vi "J1939 Workspace Tool.vi"() -> ()   [LabVIEW 2019, in "J1939 Workspace Tool.lvlib"]
uses:
  J1939 Workspace Tool.lvlib
  NationalInstruments.VeriStand.SystemStorage
  Workspace Shared/Types/UI.StateVariables.ctl
  <vilib>/NI VeriStand/Display Template Support/DisplayTemplateSupport.llb/enum_Display Template Handler Minimal To Widget Msg.ctl
  <vilib>/NI VeriStand/Execution/Workspace/SystemStateRegEventRef.ctl
  <vilib>/NI VeriStand/Execution/Workspace/Target State Info.ctl
  <vilib>/NI VeriStand/Execution/Workspace/Target State.ctl
  Shared/Types/Private Data.ctl
  <vilib>/NI/STM/TCP/TCP Connection Info.ctl
  <vilib>/NI/STM/SubVIs/MetaDataElement.ctl
  Shared/Types/Error Cluster.ctl
  Shared/Types/Error Types.ctl
  <vilib>/NI VeriStand/Display Template Support/DisplayTemplateSupport.llb/enum_Display Template Handler Minimal To Workspace.ctl
  <vilib>/NI VeriStand/Execution/Workspace/WorkspaceAPI.ctl
  <vilib>/NI VeriStand/Execution/Workspace/SystemStateEventRef.ctl
  Workspace Shared/Types/UI.Refs.ctl
  <vilib>/Utility/miscctls.llb/LVStringsAndValuesArrayTypeDef_U8.ctl
  Shared/J1939 Utilities/SubVIs/Convert CAN Arb ID to J1939 ID.vi
  <vilib>/NI VeriStand/Execution/Workspace/NI_VS Workspace ExecutionAPI.lvlib
  Shared/J1939 Utilities/J1939 Utilities.lvlib
  Shared/J1939 Addon Shared.lvlib
  <vilib>/NI/STM/NI STM.lvlib
  Workspace Shared/J1939 Workspace Shared.lvlib
  NationalInstruments.VeriStand.ClientAPI
panel:
  in  "NIVS.Workspace Event":refnum<event-registration>
  in  "NIVS.Gateway IP Address":string
  in  "NIVS.System Definition Root":refnum<k24>
  in  "Tab Control":enum32{"DTCs", "Custom RQST", "RAW FRAME"}(tab)
  in  "Refresh Continuous":bool
  in  "Clear DTC":bool
  in  "Refresh DTCs":bool
  in  "DTCs":i32(listbox)
  in  "Addresses":string(tree)
  in  "Refresh Addresses":bool
  out "Response":string
  in  "Request":bool
  in  "PGN":u32 format="%.0x"
  in  "DA":u8(ring)
  in  "Clear Array":bool
  in  "RAW":bool
  out "Priority":u8 format="%02x"
  out "SA":u8 format="%02x"
  out "PGN":u32 format="%06x"
  in  "Identifier":u32 format="%08x"
  in  "Data":u8[](array[numeric])=[0, 0, 0, 0, 0, 0, 0, 0] format="%.0x"
  out "Device":string
  in  "Errors":bool
  # "This is the root reference to the active System Definition file. You could use this to read the configuration or populate a tree with channels. You are free to close this reference, but it will be closed for you if you don't."
  # "The SystemStorageUI .NET assembly provides controls to display data configured in the System Definition file."
  # "This is the IP Address of the VeriStand Gateway to which the Workspace is connected. Use this to open all the .NET Manager references. Usually the Gateway is running on localhost, but it could be running on a neighbor's machine."
  # "This registered string User Event is used to help instruct your tool to shut down when the Workspace is closing."
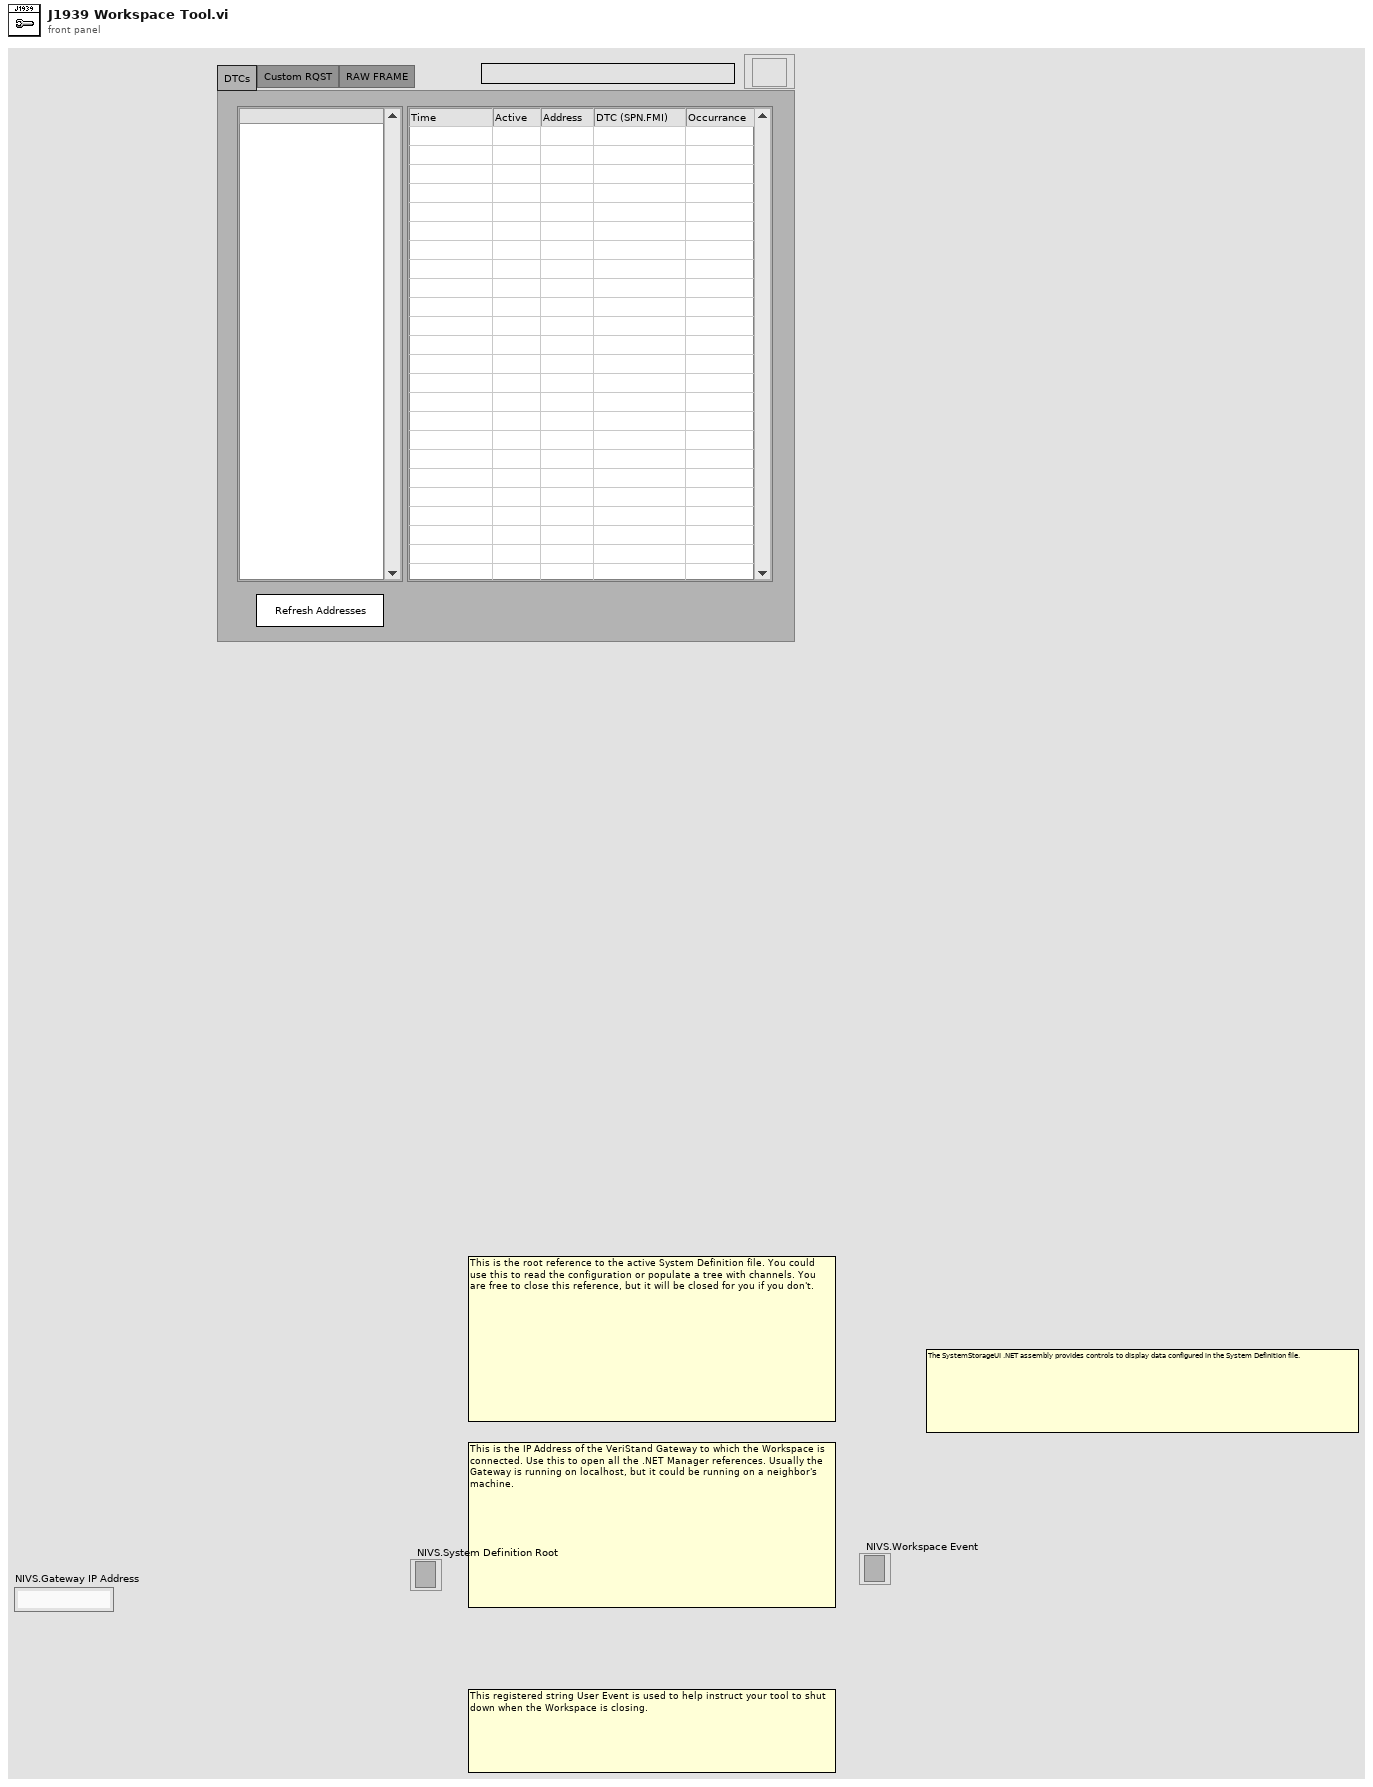
[diagram p1: front panel]
types:
  T1 = typedef "J1939 Addon Shared.lvlib/Private Data.ctl" = cluster{"PGN":u32, "DA":u8, "CD Path":string, "CD IP":string}
  T2 = typedef "J1939 Workspace Shared.lvlib/UI.StateVariables.ctl" = cluster{"NIVS.Gateway IP Address":string, "LaunchConfig.Ref":refnum<user-event>, "Events.Refs":cluster{"LaunchConfig":refnum<event-registration>, "SystemChange":T3, "NIVS.Workspace":refnum<event-registration>}, "State":T1, "TCP.Refs":T4, "Addresses.LUT":variant, "Errors.Q":refnum<queue>, "NIVS.System Definition Root":refnum<k24>, "State.Notifier":refnum<user-event>, "NIVS.Workspace.Ref":T6, "DTCs.Refresh":bool, "NIVS.State.Refs":T7, "UI.Refs":T8, "Workspace.Connected":bool, "DTCs.Timer":u32}
  T3 = typedef "NI_VS Workspace ExecutionAPI.lvlib/SystemStateRegEventRef.ctl" = refnum<event-registration>
  T4 = typedef "NI STM.lvlib/TCP Connection Info.ctl" = cluster{"connection ID":refnum<k5>, "meta data":T5[]}
  T5 = typedef "NI STM.lvlib/MetaDataElement.ctl" = string
  T6 = typedef "NI_VS Workspace ExecutionAPI.lvlib/WorkspaceAPI.ctl" = refnum<k24>
  T7 = typedef "NI_VS Workspace ExecutionAPI.lvlib/SystemStateEventRef.ctl" = cluster{"CustDatRef":refnum<user-event>, "EvtRef":refnum<k27>, "Target State User Event":refnum<user-event>}
  T8 = typedef "J1939 Workspace Shared.lvlib/UI.Refs.ctl" = cluster{"ParentVI":refnum<vi>, "DTCs":refnum<vi>, "Addresses":refnum<vi>, "Device":refnum<vi>, "Data":refnum<vi>, "Identifier":refnum<vi>, "PGN":refnum<vi>, "DA":refnum<vi>, "Refresh Continuous":refnum<vi>, "Errors":refnum<vi>, "Refresh Addresses":refnum<vi>, "Refresh DTCs":refnum<vi>, "Clear DTC":refnum<vi>, "Request":refnum<vi>, "Clear Array":refnum<vi>, "RAW":refnum<vi>}
  T9 = enum8{"Enabled", "Disabled", "Disabled and Grayed Out"}
  T10 = typedef "LVStringsAndValuesArrayTypeDef_U8.ctl" = cluster{"String":string, "Value":u8}[]
  T11 = cluster{"LaunchConfig":refnum<event-registration>, "SystemChange":T3, "NIVS.Workspace":refnum<event-registration>}
  T12 = typedef "enum_Display Template Handler Minimal To Widget Msg.ctl" = enum16{"Stop", "LaunchConfigDialog"}
  T13 = typedef "NI_VS Workspace ExecutionAPI.lvlib/SystemState.ctl" = u8
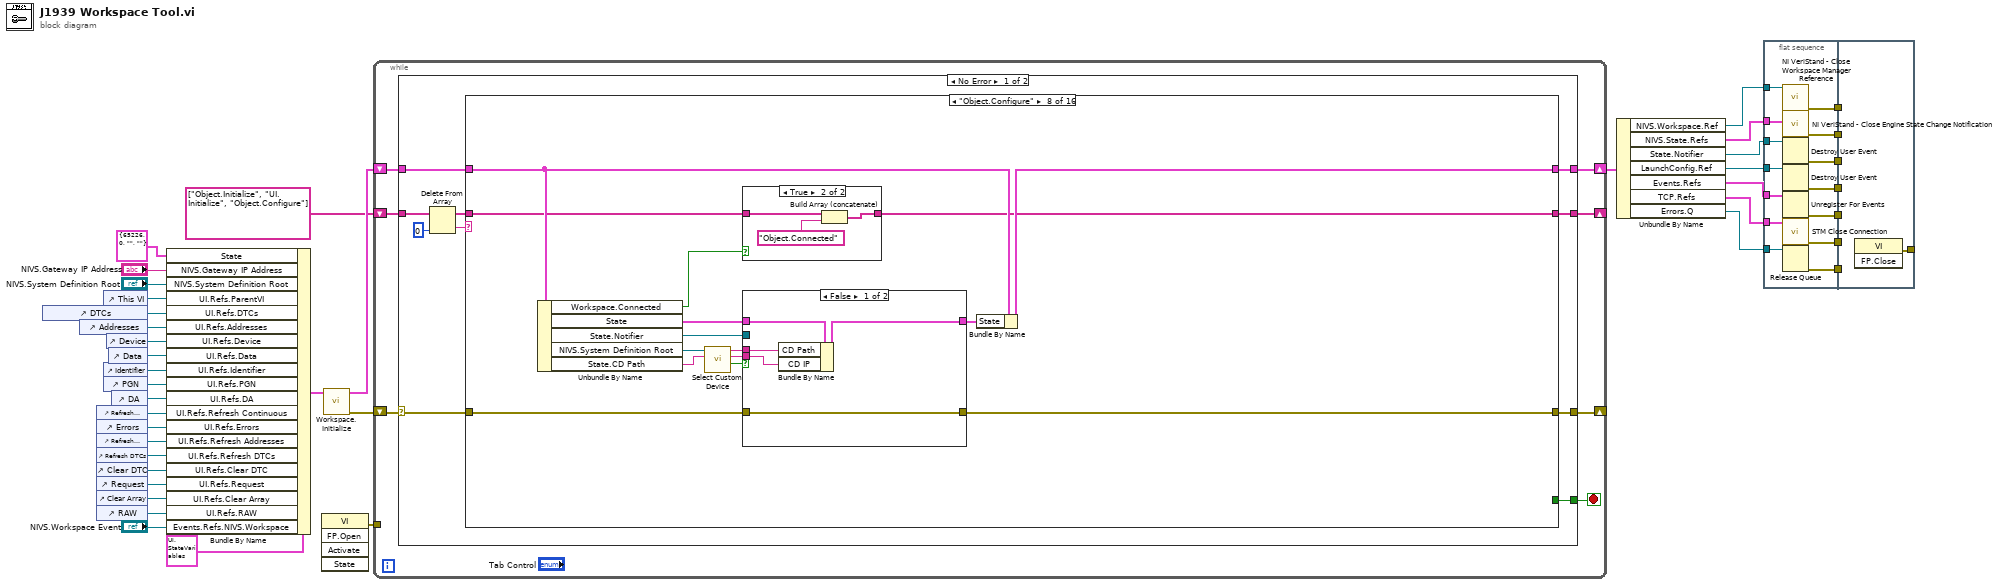
[diagram p0: block diagram]
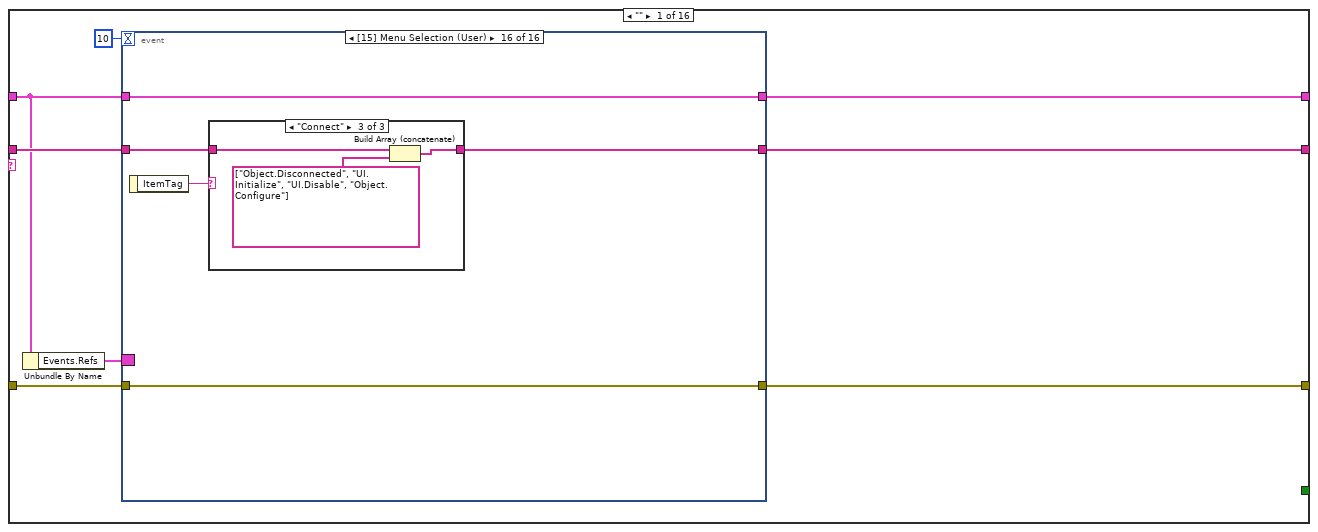
[diagram p2: hidden frame]
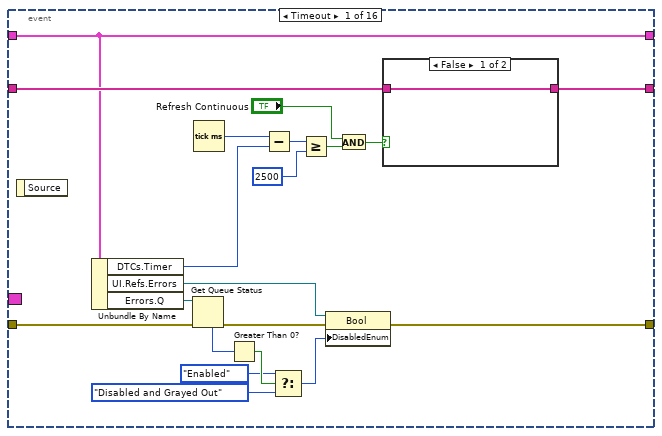
[diagram p3: hidden frame]
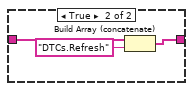
[diagram p4: hidden frame]
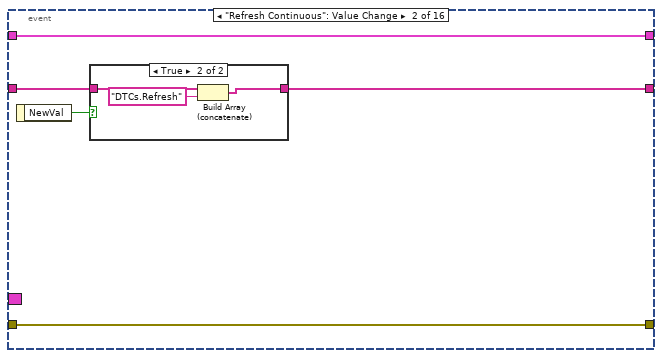
[diagram p5: hidden frame]
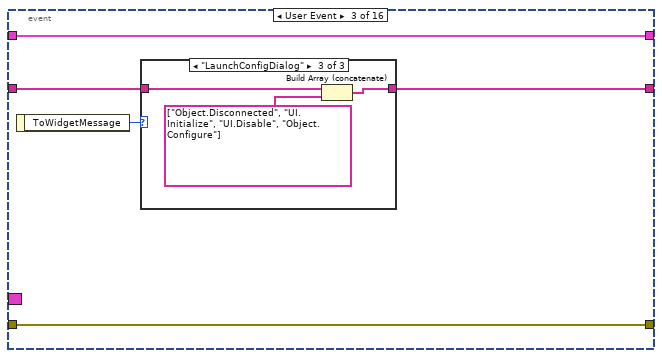
[diagram p7: hidden frame]
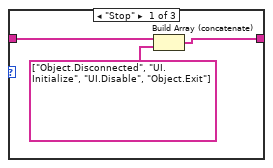
[diagram p8: hidden frame]
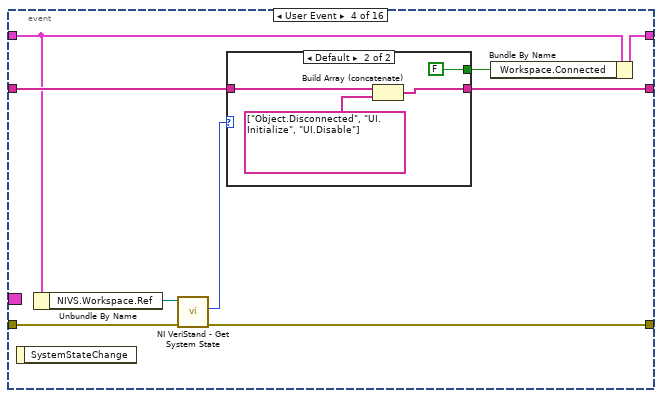
[diagram p10: hidden frame]
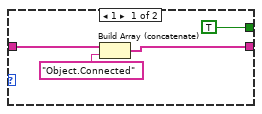
[diagram p11: hidden frame]
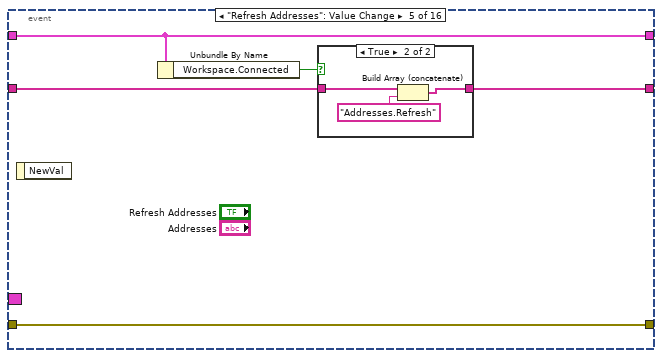
[diagram p12: hidden frame]
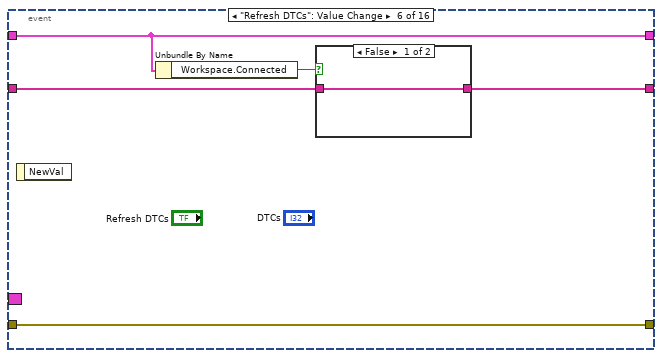
[diagram p14: hidden frame]
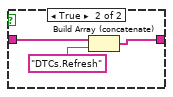
[diagram p15: hidden frame]
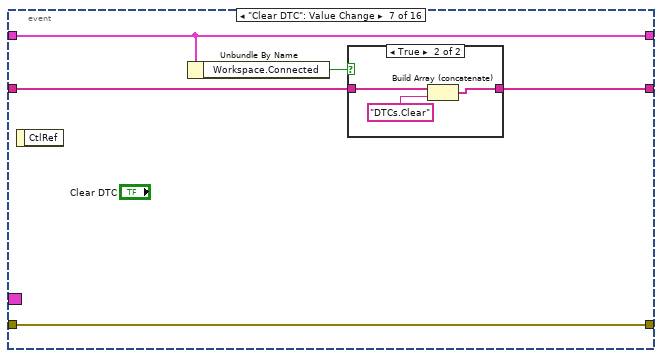
[diagram p16: hidden frame]
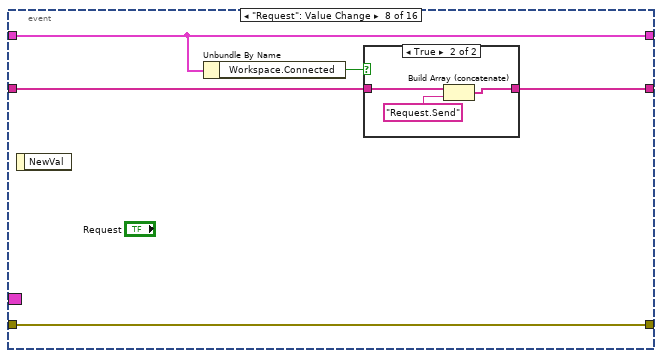
[diagram p18: hidden frame]
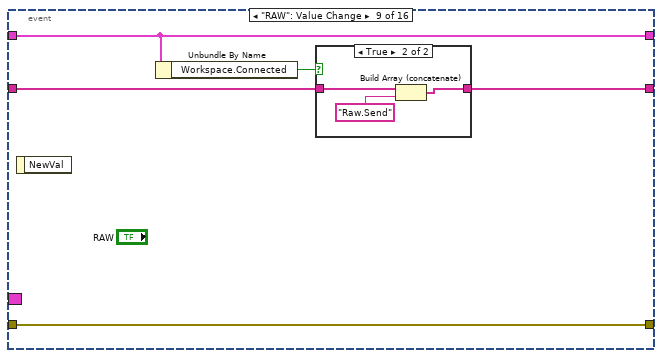
[diagram p20: hidden frame]
diagram:
  n1 = control-ref of="DTCs"() -> (w35:refnum<vi>)
  n2 = control-ref of="Addresses"() -> (w34:refnum<vi>)
  n3 = control-ref of="Refresh Continuous"() -> (w28:refnum<vi>)
  n4 = control-ref of="Errors"() -> (w27:refnum<vi>)
  n5 = control-ref of="Refresh Addresses"() -> (w26:refnum<vi>)
  n6 = control-ref of="Refresh DTCs"() -> (w25:refnum<vi>)
  n7 = control-ref of="Clear DTC"() -> (w24:refnum<vi>)
  n8 = control-ref of="Request"() -> (w23:refnum<vi>)
  n9 = control-ref of="Clear Array"() -> (w22:refnum<vi>)
  n10 = control-ref of="RAW"() -> (w21:refnum<vi>)
  n11 = control-ref of="This VI"() -> (w36:refnum<vi>)
  n12 = control-ref of="Identifier"() -> (w31:refnum<vi>)
  n13 = control-ref of="PGN"() -> (w30:refnum<vi>)
  n14 = control-ref of="Device"() -> (w33:refnum<vi>)
  n15 = control-ref of="Data"() -> (w32:refnum<vi>)
  n16 = control-ref of="DA"() -> (w29:refnum<vi>)
  n17 = Bundle By Name(cluster=T2 {"NIVS.Gateway IP Address"="", "LaunchConfig.Ref"=refnum, "Events.Refs"={"LaunchConfig"=refnum, "SystemChange"=refnum, "NIVS.Workspace"=refnum}, "State"={"PGN"=0, "DA"=0, "CD Path"="", "CD IP"=""}, "TCP.Refs"={"connection ID"=refnum, "meta data"=[]}, "Addresses.LUT"=variant, "Errors.Q"=refnum, "NIVS.System Definition Root"=refnum, "State.Notifier"=refnum, "NIVS.Workspace.Ref"=refnum, "DTCs.Refresh"=FALSE, "NIVS.State.Refs"={"CustDatRef"=refnum, "EvtRef"=refnum, "Target State User Event"=refnum}, "UI.Refs"={"ParentVI"=refnum, "DTCs"=refnum, "Addresses"=refnum, "Device"=refnum, "Data"=refnum, "Identifier"=refnum, "PGN"=refnum, "DA"=refnum, "Refresh Continuous"=refnum, "Errors"=refnum, "Refresh Addresses"=refnum, "Refresh DTCs"=refnum, "Clear DTC"=refnum, "Request"=refnum, "Clear Array"=refnum, "RAW"=refnum}, "Workspace.Connected"=FALSE, "DTCs.Timer"=0}, "State"=T1 {"PGN"=65226, "DA"=0, "CD Path"="", "CD IP"=""} ("Cluster"), "NIVS.Gateway IP Address"="NIVS.Gateway IP Address", "NIVS.System Definition Root"="NIVS.System Definition Root", "UI.Refs.ParentVI"=w36, "UI.Refs.DTCs"=w35, "UI.Refs.Addresses"=w34, "UI.Refs.Device"=w33, "UI.Refs.Data"=w32, "UI.Refs.Identifier"=w31, "UI.Refs.PGN"=w30, "UI.Refs.DA"=w29, "UI.Refs.Refresh Continuous"=w28, "UI.Refs.Errors"=w27, "UI.Refs.Refresh Addresses"=w26, "UI.Refs.Refresh DTCs"=w25, "UI.Refs.Clear DTC"=w24, "UI.Refs.Request"=w23, "UI.Refs.Clear Array"=w22, "UI.Refs.RAW"=w21, "Events.Refs.NIVS.Workspace"="NIVS.Workspace Event") -> (w38:T2)
  n18 = invoke class="VI" method="FP.Open"() -> (error out=w8:errorcluster)  [unwired: 5 in, 4 out]
  n19 = call "Workspace.Initialize.vi"("State"=w38) -> ("error out"=w37:errorcluster, "State"=w20:T2)  [unwired: 9 in]
  n20 = while {
    shift-right: [w46] -> _
    shift-left: w37 -> [w47]
    shift-right: [w42] -> w18
    shift-left: w20 -> [w45]
    shift-right: [w43] -> _
    shift-left: string[] ["Object.Initialize", "UI.Initialize", "Object.Configure"] -> [w44]
    tunnel: w8 -> [_]
    stop <- w48 stop-if-true
    n21 = case shown="No Error" w47 {
      selector: w47 -> [w49 w503]
      tunnel: [w58 FALSE] -> w48
      tunnel: [w50 w501] -> w46
      tunnel: w45 -> [w57 w498]
      tunnel: w44 -> [w55 w499]
      tunnel: [w52 w499] -> w43
      tunnel: [w51 w498] -> w42
      frame No Error {
        n22 = Delete From Array(array=w55, index=0) -> (deleted portion=w54:string, array with subset deleted=w53:string[])  [unwired: 1 in]
        n23 = case shown="\"Object.Configure\"" w54 {
          selector: w54 -> [_ _ _ _ _ _ _ _ _ _ _ _ _ _ _ w493]
          tunnel: [_ _ _ _ _ _ _ _ TRUE _ _ _ _ _ _ _] -> w58
          tunnel: w57 -> [w60 w232 w241 w258 w288 w324 w337 w357 w381 w390 w398 w410 w419 w440 w488 w496]
          tunnel: w53 -> [w64 w239 w251 w267 w295 w316 w340 w354 w382 w391 w399 w406 w435 w456 w490 w497]
          tunnel: [w65 w239 w251 w267 w294 w316 w339 w353 w382 w391 w399 w406 w435 w456 w490 w497] -> w52
          tunnel: [w63 w229 w240 w268 w287 w323 w336 w356 w381 w390 w397 w407 w419 w440 w488 w496] -> w51
          tunnel: [w62 w228 w250 w253 w290 w318 w335 w360 w380 w386 w392 w405 w420 w441 w464 w495] -> w50
          tunnel: w49 -> [w61 w228 w250 w254 w289 w319 w325 w361 w380 w385 w392 w405 w422 w443 w489 w495]
          frame "" {
            n24 = Unbundle By Name(w60) -> ("Events.Refs"=w59:T11)
            n25 = event shown="[15] Menu Selection (User)" {
              selector: w59 -> [_ _ _ _ _ _ _ _ _ _ _ _ _ _ _ _]
              dyn-events: _ -> [_ _ _ _ _ _ _ _ _ _ _ _ _ _ _ _]
              timeout: 10 -> [_ _ _ _ _ _ _ _ _ _ _ _ _ _ _ _]
              tunnel: w60 -> [w75 w94 w104 w114 w132 w140 w147 w158 w167 w176 w185 w189 w196 w206 w211 w220]
              tunnel: [w76 w92 w100 w117 w130 w138 w148 w156 w165 w174 w184 w190 w198 w201 w208 w216] -> w65
              tunnel: w64 -> [w77 w93 w101 w118 w131 w139 w149 w157 w166 w175 w187 w190 w198 w202 w209 w218]
              tunnel: [w75 w94 w104 w113 w132 w140 w147 w158 w167 w176 w185 w189 w196 w206 w211 w220] -> w63
              tunnel: [w69 w95 w103 w119 w133 w142 w151 w160 w169 w178 w186 w188 w197 w205 w210 w219] -> w62
              tunnel: w61 -> [w71 w95 w103 w120 w133 w142 w151 w160 w169 w178 w186 w188 w197 w205 w210 w219]
              event Timeout {
                n26 = event-data() -> ()  [unwired: 2 out]
                n27 = Unbundle By Name(w75) -> ("DTCs.Timer"=w68:u32, "UI.Refs.Errors"=w73:refnum<vi>, "Errors.Q"=w74:refnum<queue>)
                n28 = Get Queue Status(queue=w74, error in (no error)=w71) -> (error out=w72:errorcluster, # elements in queue=w86:i32)  [unwired: 1 in, 6 out]
                n29 = Tick Count (ms)() -> (millisecond timer value=w80:u32)
                n30 = Greater Than 0?(x=w86) -> (x > 0?=w85:bool)
                n31 = Subtract(x=w80, y=w68) -> (x-y=w82:u32)
                n32 = Select(t=T9."Enabled" ("Disabled"), s=w85, f=T9."Disabled and Grayed Out") -> (s? t:f=w70:T9)
                n33 = Greater Or Equal?(x=w82, y=u32 2500) -> (x >= y?=w67:bool)
                n34 = property class="Bool"(reference=w73, error in=w72, "DisabledEnum"=w70) -> (error out=w69:errorcluster)  [unwired: 1 out]
                n35 = And(x="Refresh Continuous", y=w67) -> (x .and. y?=w78:bool)
                n36 = case shown="False" w78 {
                  tunnel: w77 -> [w87 w89]
                  tunnel: [w87 w88] -> w76
                  frame False {
                  }
                  frame True {
                    n37 = Build Array (concatenate)(w89, "DTCs.Refresh" ("NewVal")) -> (w88:string[])
                  }
                }
              }
              event "Refresh Continuous": Value Change {
                n38 = event-data() -> ("NewVal"=w91:bool)  [unwired: 1 out]
                n39 = case shown="True" w91 {
                  tunnel: w93 -> [w96 w98]
                  tunnel: [w96 w97] -> w92
                  frame False {
                  }
                  frame True {
                    n40 = Build Array (concatenate)(w98, "DTCs.Refresh" ("NewVal")) -> (w97:string[])
                  }
                }
              }
              event User Event {
                n41 = event-data() -> ("ToWidgetMessage"=w102:T12)  [unwired: 1 out]
                n42 = case shown="\"LaunchConfigDialog\"" w102 {
                  tunnel: w101 -> [w106 w108 w110]
                  tunnel: [w105 w108 w109] -> w100
                  frame "Stop" {
                    n43 = Build Array (concatenate)(w106, string[] ["Object.Disconnected", "UI.Initialize", "UI.Disable", "Object.Exit"]) -> (w105:string[])
                  }
                  frame Default {
                  }
                  frame "LaunchConfigDialog" {
                    n44 = Build Array (concatenate)(w110, string[] ["Object.Disconnected", "UI.Initialize", "UI.Disable", "Object.Configure"]) -> (w109:string[])
                  }
                }
              }
              event User Event {
                n45 = event-data() -> ()  [unwired: 2 out]
                n46 = Unbundle By Name(w114) -> ("NIVS.Workspace.Ref"=w115:T6)
                n47 = call <vilib>:"NI VeriStand - Get System State.vi"("error in (no error)"=w120, "WorkspaceManager in"=w115) -> ("error out"=w119:errorcluster, "System State"=w116:T13)  [unwired: 5 in, 3 out]
                n48 = case shown="Default" w116 {
                  tunnel: w118 -> [w124 w128]
                  tunnel: [w123 w127] -> w117
                  tunnel: [TRUE FALSE] -> w112
                  frame 1 {
                    # "System state is connected"
                    n49 = Build Array (concatenate)(w124, "Object.Connected") -> (w123:string[])
                  }
                  frame Default {
                    # "System state not connected"
                    n50 = Build Array (concatenate)(w128, string[] ["Object.Disconnected", "UI.Initialize", "UI.Disable"]) -> (w127:string[])
                  }
                }
                n51 = Bundle By Name(cluster=w114, "Workspace.Connected"=w112) -> (w113:T2)
              }
              event "Refresh Addresses": Value Change {
                n52 = event-data() -> ()  [unwired: 2 out]
                n53 = Unbundle By Name(w132) -> ("Workspace.Connected"=w129:bool)
                n54 = case shown="True" w129 {
                  tunnel: w131 -> [w134 w136]
                  tunnel: [w134 w135] -> w130
                  frame False {
                  }
                  frame True {
                    n55 = Build Array (concatenate)(w136, "Addresses.Refresh") -> (w135:string[])
                  }
                }
              }
              event "Refresh DTCs": Value Change {
                n56 = event-data() -> ()  [unwired: 2 out]
                n57 = Unbundle By Name(w140) -> ("Workspace.Connected"=w141:bool)
                n58 = case shown="False" w141 {
                  tunnel: w139 -> [w143 w145]
                  tunnel: [w143 w144] -> w138
                  frame False {
                  }
                  frame True {
                    n59 = Build Array (concatenate)(w145, "DTCs.Refresh") -> (w144:string[])
                  }
                }
              }
              event "Clear DTC": Value Change {
                n60 = event-data() -> ()  [unwired: 2 out]
                n61 = Unbundle By Name(w147) -> ("Workspace.Connected"=w150:bool)
                n62 = case shown="True" w150 {
                  tunnel: w149 -> [w152 w154]
                  tunnel: [w152 w153] -> w148
                  frame False {
                  }
                  frame True {
                    n63 = Build Array (concatenate)(w154, "DTCs.Clear") -> (w153:string[])
                  }
                }
              }
              event "Request": Value Change {
                n64 = event-data() -> ()  [unwired: 2 out]
                n65 = Unbundle By Name(w158) -> ("Workspace.Connected"=w159:bool)
                n66 = case shown="True" w159 {
                  tunnel: w157 -> [w161 w163]
                  tunnel: [w161 w162] -> w156
                  frame False {
                  }
                  frame True {
                    n67 = Build Array (concatenate)(w163, "Request.Send") -> (w162:string[])
                  }
                }
              }
              event "RAW": Value Change {
                n68 = event-data() -> ()  [unwired: 2 out]
                n69 = Unbundle By Name(w167) -> ("Workspace.Connected"=w168:bool)
                n70 = case shown="True" w168 {
                  tunnel: w166 -> [w170 w172]
                  tunnel: [w170 w171] -> w165
                  frame False {
                  }
                  frame True {
                    n71 = Build Array (concatenate)(w172, "Raw.Send") -> (w171:string[])
                  }
                }
              }
              event "Clear Array": Value Change {
                n72 = event-data() -> ()  [unwired: 2 out]
                n73 = Unbundle By Name(w176) -> ("Workspace.Connected"=w177:bool)
                n74 = case shown="True" w177 {
                  tunnel: w175 -> [w179 w181]
                  tunnel: [w179 w180] -> w174
                  frame False {
                  }
                  frame True {
                    n75 = Build Array (concatenate)(w181, "Raw.Clear") -> (w180:string[])
                  }
                }
              }
              event "Addresses": Value Change {
                n76 = event-data() -> ()  [unwired: 2 out]
                n77 = Build Array (concatenate)(w187, "DTCs.Refresh" ("NewVal")) -> (w184:string[])
              }
              event "Identifier": Value Change {
                n78 = event-data() -> ("NewVal"=w191:u32)  [unwired: 1 out]
                n79 = call-poly "Common Conversions.vi"("Arb ID"=w191) -> ("Priority"=→"Priority":u8, "PGN"=→"PGN":u32, "Source Address"=→"SA":u8)  [unwired: 11 in, 1 out]
              }
              event "Errors": Value Change {
                n80 = event-data() -> ()  [unwired: 2 out]
                n81 = Unbundle By Name(w196) -> ("Errors.Q"=w195:refnum<queue>)
                n82 = flat-sequence {
                  tunnel: [w200] -> w199
                  tunnel: w195 -> [w200]
                  frame #0 {
                  }
                }
                n83 = call "Error Display.vi"("queue out"=w199) -> ()  [unwired: 11 in]
              }
              event Panel Close? {
                n84 = event-data() -> ()  [unwired: 5 out]
                n85 = Build Array (concatenate)(w202, string[] ["Object.Disconnected", "UI.Initialize", "UI.Disable", "Object.Exit"]) -> (w201:string[])
                n86 = event-data("Discard?"=TRUE) -> ()  [unwired: 1 in, 1 out]
              }
              event User Event {
                n87 = event-data() -> ("Workspace Event"=w207:string)  [unwired: 1 out]
                n88 = case shown="\"Disconnect\", \"Shut Down\"" w207 {
                  tunnel: w209 -> [w212 w214]
                  tunnel: [w212 w213] -> w208
                  frame Default {
                  }
                  frame "Disconnect", "Shut Down" {
                    n89 = Build Array (concatenate)(w214, string[] ["Object.Disconnected", "UI.Initialize", "UI.Disable", "Object.Exit"]) -> (w213:string[])
                  }
                }
              }
              event Menu Selection (User) {
                n90 = event-data() -> ("ItemTag"=w217:string)  [unwired: 1 out]
                n91 = case shown="\"Connect\"" w217 {
                  tunnel: w218 -> [w222 w224 w226]
                  tunnel: [w221 w224 w225] -> w216
                  frame "Exit" {
                    n92 = Build Array (concatenate)(w222, string[] ["Object.Disconnected", "UI.Initialize", "UI.Disable", "Object.Exit"]) -> (w221:string[])
                  }
                  frame Default {
                  }
                  frame "Connect" {
                    n93 = Build Array (concatenate)(w226, string[] ["Object.Disconnected", "UI.Initialize", "UI.Disable", "Object.Configure"]) -> (w225:string[])
                  }
                }
              }
            }
          }
          frame "Addresses.Refresh" {
            n94 = Unbundle By Name(w232) -> ("UI.Refs.Addresses"=w238:refnum<vi>, "UI.Refs.DA"=w237:refnum<vi>, "TCP.Refs"=w236:T4, "State"=w235:T1, "Errors.Q"=w234:refnum<queue>, "UI.Refs.ParentVI"=w233:refnum<vi>)
            n95 = call "Request Addresses Event.vi"("connection info"=w236, "DA"=w237, "Addresses"=w238, "State Variables"=w235, "Error Q"=w234, "VI Ref"=w233) -> ("connection info"=w231:T4, "Address Lookup Table Out"=w230:variant)  [unwired: 8 in]
            n96 = Bundle By Name(cluster=w232, "TCP.Refs"=w231, "Addresses.LUT"=w230) -> (w229:T2)
          }
          frame "DTCs.Clear" {
            n97 = Unbundle By Name(w241) -> ("UI.Refs.Addresses"=w244:refnum<vi>, "TCP.Refs"=w249:T4, "State"=w248:T1, "Addresses.LUT"=w247:variant, "Errors.Q"=w246:refnum<queue>, "UI.Refs.ParentVI"=w245:refnum<vi>)
            n98 = call "Clear DTCs Event.vi"("connection info"=w249, "Addresses"=w244, "State Variables"=w248, "Address Lookup Table"=w247, "Error Q"=w246, "VI Ref"=w245) -> ("connection info"=w243:T4, "Address Lookup Table Out"=w242:variant)  [unwired: 8 in]
            n99 = Bundle By Name(cluster=w241, "TCP.Refs"=w243, "Addresses.LUT"=w242) -> (w240:T2)
          }
          frame "DTCs.Refresh" {
            n100 = Unbundle By Name(w258) -> ("UI.Refs.DTCs"=w265:refnum<vi>, "UI.Refs.Addresses"=w264:refnum<vi>, "TCP.Refs"=w263:T4, "State"=w262:T1, "Addresses.LUT"=w261:variant, "Errors.Q"=w260:refnum<queue>, "UI.Refs.ParentVI"=w259:refnum<vi>, "UI.Refs.Refresh Continuous"=w255:refnum<vi>)
            n101 = property class="Bool (strict)"(reference=w255, error in=w254) -> (error out=w253:errorcluster, "Value"=w252:bool)  [unwired: 1 out]
            n102 = Not(x=w252) -> (.not. x?=w266:bool)
            n103 = flat-sequence {
              tunnel: w261 -> [w281]
              tunnel: w263 -> [w279]
              tunnel: w262 -> [w277]
              tunnel: w266 -> [w276]
              tunnel: [w280] -> w271
              tunnel: [w278] -> w270
              tunnel: w265 -> [w275]
              tunnel: w264 -> [w274]
              tunnel: w260 -> [w273]
              tunnel: w259 -> [w272]
              tunnel: [w283] -> w256
              tunnel: [w284] -> w257
              tunnel: w271 -> [w284]
              tunnel: w270 -> [w283]
              tunnel: [w282] -> w269
              frame #0 {
                n104 = call "Refresh DTCs Event.vi"("connection info"=w279, "Addresses"=w274, "DTCs"=w275, "State Variables"=w277, "Address Lookup Table"=w281, "To Top (T)"=w276, "Error Q"=w273, "VI Ref"=w272) -> ("connection info"=w278:T4, "Address Lookup Table Out"=w280:variant)  [unwired: 6 in]
              }
              frame #1 {
                n105 = Tick Count (ms)() -> (millisecond timer value=w282:u32)
              }
            }
            n106 = Bundle By Name(cluster=w258, "DTCs.Timer"=w269, "TCP.Refs"=w256, "Addresses.LUT"=w257) -> (w268:T2)
          }
          frame "Object.Connected" {
            n107 = Unbundle By Name(w288) -> ("TCP.Refs"=w286:T4, "State.CD IP"=w291:string, "State.CD Path"=w292:string)
            n108 = call "STM Close Connection.vi"("connection info"=w286) -> ("error out"=w285:errorcluster)  [unwired: 10 in]
            n109 = flat-sequence {
              tunnel: w295 -> [w309]
              tunnel: [w307] -> w294
              tunnel: "/Custom Devices/" ("regular expression") -> [w306]
              tunnel: w292 -> [w305]
              tunnel: w291 -> [w304]
              tunnel: [w302] -> w290
              tunnel: w289 -> [w301]
              tunnel: w288 -> [w299]
              tunnel: [w298] -> w287
              tunnel: w285 -> [_]
              frame #0 {
                n110 = Match Pattern(string=w305, regular expression=w306) -> (after substring=w296:string)  [unwired: 1 in, 3 out]
                n111 = call "Open Connection to Target.vi"("error in (no error)"=w301, "IP Address"=w304, "TCP Service"=w296) -> ("error out"=w303:errorcluster, "connection info"=w300:T4)  [unwired: 7 in]
                n112 = Bundle By Name(cluster=w299, "TCP.Refs"=w300) -> (w298:T2)
                n113 = case shown="No Error" w303 {
                  selector: w303 -> [w311 w315]
                  tunnel: [string[] ["UI.Enable"] ("element") string[] ["UI.Initialize", "UI.Disable"] ("element")] -> w308
                  tunnel: [w311 w315] -> w302
                  tunnel: [w310 "Not Connected" ("CD Path")] -> w297
                  tunnel: w296 -> [w310 _]
                  frame No Error {
                  }
                  frame Error {
                  }
                }
                "Device" <- w297
                n114 = Build Array (concatenate)(w309, w308) -> (w307:string[])
              }
            }
          }
          frame "Object.Disconnected" {
            n115 = Unbundle By Name(w324) -> ("TCP.Refs"=w322:T4, "UI.Refs.Device"=w320:refnum<vi>)
            n116 = Bundle By Name(cluster=w324, "TCP.Refs"=T4 {"connection ID"=refnum, "meta data"=[]}) -> (w323:T2)
            n117 = property class="Str"(reference=w320, error in=w319, "Value"="Not Connected") -> (error out=w318:errorcluster)  [unwired: 1 out]
            n118 = call "STM Close Connection.vi"("connection info"=w322) -> ()  [unwired: 10 in, 1 out]
          }
          frame "Object.Initialize" {
            n119 = Unbundle By Name(w337) -> ("State.CD IP"=w333:string, "State.CD Path"=w332:string, "NIVS.Workspace.Ref"=w341:T6)
            n120 = Empty String/Path?(string/path=w333) -> (empty?=w331:bool)
            n121 = Empty String/Path?(string/path=w332) -> (empty?=w330:bool)
            n122 = Compound Arithmetic op=OR(w331, w330) -> (w328:bool)
            n123 = Build Array("Object.Connected") -> (w326:string[])
            n124 = call <vilib>:"NI VeriStand - Get System State.vi"("error in (no error)"=w325, "WorkspaceManager in"=w341) -> ("error out"=w335:errorcluster, "System State"=w334:T13)  [unwired: 5 in, 3 out]
            n125 = case shown="1" w334 {
              tunnel: w340 -> [w348 w352]
              tunnel: [w347 w351] -> w339
              tunnel: [TRUE FALSE] -> w338
              tunnel: string[] ["Object.Disconnected", "UI.Initialize", "UI.Disable"] -> [w344 w349]
              tunnel: w328 -> [w345 _]
              tunnel: w326 -> [w342 _]
              frame 1 {
                n126 = Select(t=w344, s=w345, f=w342) -> (s? t:f=w343:string[])
                n127 = Build Array (concatenate)(w348, w343) -> (w347:string[])
              }
              frame Default {
                n128 = Build Array (concatenate)(w352, w349) -> (w351:string[])
              }
            }
            n129 = Bundle By Name(cluster=w337, "Workspace.Connected"=w338) -> (w336:T2)
          }
          frame "Object.Configure" {
            n130 = Unbundle By Name(w357) -> ("Workspace.Connected"=w355:bool, "State"=w359:T1, "State.Notifier"=w362:refnum<user-event>, "NIVS.System Definition Root"=w363:refnum<k24>, "State.CD Path"=w366:string)
            n131 = call "Select Custom Device.vi"("CD Path"=w366, "NIVS.System Definition Root"=w363) -> ("Cancelled?"=w364:bool, "IP Address"=w367:string, "Custom Device Path Out"=w365:string)  [unwired: 7 in]
            n132 = case shown="True" w355 {
              tunnel: w354 -> [w368 w371]
              tunnel: [w368 w369] -> w353
              frame False {
              }
              frame True {
                n133 = Build Array (concatenate)(w371, "Object.Connected") -> (w369:string[])
              }
            }
            n134 = case shown="False" w364 {
              tunnel: w362 -> [_ _]
              tunnel: w367 -> [w375 _]
              tunnel: w365 -> [w376 _]
              tunnel: w361 -> [w372 w378]
              tunnel: [w372 w378] -> w360
              tunnel: w359 -> [w374 w377]
              tunnel: [w373 w377] -> w358
              frame False {
                n135 = Bundle By Name(cluster=w374, "CD Path"=w376, "CD IP"=w375) -> (w373:T1)
              }
              frame True {
              }
            }
            n136 = Bundle By Name(cluster=w357, "State"=w358) -> (w356:T2)
          }
          frame "Object.Exit" {
          }
          frame "Raw.Clear" {
            n137 = Unbundle By Name(w390) -> ("UI.Refs.Identifier"=w388:refnum<vi>, "UI.Refs.Data"=w389:refnum<vi>)
            n138 = property class="Arr (strict)"(reference=w389, error in=w385, "Value"=u8[] []) -> (error out=w387:errorcluster)  [unwired: 1 out]
            n139 = property class="DigNum (strict)"(reference=w388, error in=w387, "Val(Sgnl)"=u32 0 ("Value (Signaling)")) -> (error out=w386:errorcluster)  [unwired: 1 out]
          }
          frame "Raw.Send" {
            n140 = Unbundle By Name(w398) -> ("TCP.Refs"=w402:T4, "State"=w401:T1, "Addresses.LUT"=w400:variant, "Errors.Q"=w396:refnum<queue>, "UI.Refs.ParentVI"=w395:refnum<vi>)
            n141 = call "RAW Event.vi"("connection info"=w402, "State Variables"=w401, "Address Lookup Table"=w400, "Identifier"="Identifier", "Data"="Data", "Error Q"=w396, "VI Ref"=w395) -> ("connection info"=w394:T4, "Address Lookup Table Out"=w393:variant)  [unwired: 7 in]
            n142 = Bundle By Name(cluster=w398, "TCP.Refs"=w394, "Addresses.LUT"=w393) -> (w397:T2)
          }
          frame "Request.Send" {
            n143 = Unbundle By Name(w410) -> ("TCP.Refs"=w415:T4, "State"=w414:T1, "Addresses.LUT"=w413:variant, "Errors.Q"=w412:refnum<queue>, "UI.Refs.ParentVI"=w411:refnum<vi>)
            n144 = call "Request Event.vi"("connection info"=w415, "State Variables"=w414, "Address Lookup Table"=w413, "PGN"="PGN", "DA"="DA", "Error Q"=w412, "VI Ref"=w411) -> ("connection info"=w409:T4, "Response"=→"Response":string, "Address Lookup Table Out"=w408:variant)  [unwired: 6 in]
            n145 = Bundle By Name(cluster=w410, "TCP.Refs"=w409, "Addresses.LUT"=w408) -> (w407:T2)
          }
          frame "UI.Disable" {
            n146 = Unbundle By Name(w419) -> ("UI.Refs.Data"=w434:refnum<vi>, "UI.Refs.Identifier"=w433:refnum<vi>, "UI.Refs.PGN"=w432:refnum<vi>, "UI.Refs.DA"=w431:refnum<vi>, "UI.Refs.Refresh Continuous"=w430:refnum<vi>, "UI.Refs.Errors"=w429:refnum<vi>, "UI.Refs.Refresh Addresses"=w428:refnum<vi>, "UI.Refs.Refresh DTCs"=w427:refnum<vi>, "UI.Refs.Clear DTC"=w426:refnum<vi>, "UI.Refs.Request"=w425:refnum<vi>, "UI.Refs.Clear Array"=w424:refnum<vi>, "UI.Refs.RAW"=w423:refnum<vi>)
            n147 = Build Array(w434, w433, w432, w431, w430, w429, w428, w427, w426, w425, w424, w423) -> (w421:refnum<vi>[])
            n148 = for {
              shift-right: [w437] -> w420
              shift-left: w422 -> [w439]
              tunnel: w421 -> [w438] mode=indexing
              n149 = property class="Ctl"(reference=w438, error in=w439, "DisabledEnum"=T9."Disabled and Grayed Out" ("Disabled")) -> (error out=w437:errorcluster)  [unwired: 1 out]
            }
          }
          frame "UI.Enable" {
            n150 = Unbundle By Name(w440) -> ("UI.Refs.Data"=w455:refnum<vi>, "UI.Refs.Identifier"=w454:refnum<vi>, "UI.Refs.PGN"=w453:refnum<vi>, "UI.Refs.DA"=w452:refnum<vi>, "UI.Refs.Refresh Continuous"=w451:refnum<vi>, "UI.Refs.Errors"=w450:refnum<vi>, "UI.Refs.Refresh Addresses"=w449:refnum<vi>, "UI.Refs.Refresh DTCs"=w448:refnum<vi>, "UI.Refs.Clear DTC"=w447:refnum<vi>, "UI.Refs.Request"=w446:refnum<vi>, "UI.Refs.Clear Array"=w445:refnum<vi>, "UI.Refs.RAW"=w444:refnum<vi>)
            n151 = Build Array(w455, w454, w453, w452, w451, w450, w449, w448, w447, w446, w445, w444) -> (w442:refnum<vi>[])
            n152 = for {
              shift-right: [w458] -> w441
              shift-left: w443 -> [w460]
              tunnel: w442 -> [w459] mode=indexing
              n153 = property class="Ctl"(reference=w459, error in=w460, "DisabledEnum"=T9."Enabled" ("Disabled")) -> (error out=w458:errorcluster)  [unwired: 1 out]
            }
          }
          frame "UI.Initialize" {
            (unwired) FALSE ("Value")
            n154 = Unbundle By Name(w488) -> ("UI.Refs.Errors"=w462:refnum<vi>, "UI.Refs.Data"=w469:refnum<vi>, "UI.Refs.Identifier"=w473:refnum<vi>, "UI.Refs.DA"=w475:refnum<vi>, "UI.Refs.PGN"=w478:refnum<vi>, "UI.Refs.DTCs"=w481:refnum<vi>, "UI.Refs.Addresses"=w484:refnum<vi>, "UI.Refs.Refresh Continuous"=w485:refnum<vi>, "UI.Refs.Device"=w486:refnum<vi>)
            n155 = property class="Str"(reference=w486, error in=w489, "Value"="Not Connected") -> (error out=w491:errorcluster)  [unwired: 1 out]
            n156 = property class="Bool (strict)"(reference=w485, error in=w491, "Value"=FALSE) -> (error out=w482:errorcluster)  [unwired: 1 out]
            n157 = invoke class="Tree (strict)" method="Edit Tree Items.Delete"(reference=w484, error in=w482, "Delete Children"=TRUE ("Delete Children?")) -> (error out=w479:errorcluster)  [unwired: 2 in, 4 out]
            n158 = property class="MCListbox (strict)"(reference=w481, error in=w479, "ItemNames"=string[][] [] ("Item Names")) -> (error out=w476:errorcluster)  [unwired: 1 out]
            n159 = property class="DigNum (strict)"(reference=w478, error in=w476, "Value"=u32 0) -> (error out=w474:errorcluster)  [unwired: 1 out]
            n160 = property class="Ring (strict)"(reference=w475, error in=w474, "Value"=u8 0, "StringsAndValues[]"=T10 [] ("Strings And Values []")) -> (error out=w472:errorcluster)  [unwired: 1 out]
            n161 = property class="DigNum (strict)"(reference=w473, error in=w472, "Val(Sgnl)"=u32 0 ("Value (Signaling)")) -> (error out=w468:errorcluster)  [unwired: 1 out]
            n162 = property class="Arr (strict)"(reference=w469, error in=w468, "Value"=u8[] []) -> (error out=w465:errorcluster)  [unwired: 1 out]
            n163 = property class="Bool"(reference=w462, error in=w465, "DisabledEnum"=T9."Disabled and Grayed Out" ("f")) -> (error out=w464:errorcluster)  [unwired: 1 out]
          }
          frame Default {
            n164 = Concatenate Strings(w493, " is not a valid command." ("string")) -> (w492:string)
            n165 = One Button Dialog(message=w492) -> ()  [unwired: 1 in, 1 out]
          }
        }
      }
      frame Error {
        n166 = call <vilib>:"Simple Error Handler.vi"("error in (no error)"=w503) -> ("error out"=w502:errorcluster)  [unwired: 4 in, 4 out]
        n167 = call <vilib>:"Clear Errors.vi"("error in (no error)"=w502) -> ("error out"=w501:errorcluster)  [unwired: 5 in, 1 out]
      }
    }
  }
  n168 = Unbundle By Name(w18) -> ("NIVS.Workspace.Ref"=w13:T6, "NIVS.State.Refs"=w14:T7, "State.Notifier"=w16:refnum<user-event>, "LaunchConfig.Ref"=w17:refnum<user-event>, "Events.Refs"=w15:T11, "TCP.Refs"=w12:T4, "Errors.Q"=w9:refnum<queue>)
  n169 = flat-sequence {
    tunnel: w17 -> [w517]
    tunnel: w16 -> [w516]
    tunnel: w15 -> [w515]
    tunnel: w14 -> [w514]
    tunnel: w13 -> [w513]
    tunnel: w12 -> [w507]
    tunnel: w9 -> [w504]
    tunnel: [w512] -> w7
    tunnel: [w511] -> w6
    tunnel: [w510] -> w5
    tunnel: [w509] -> w4
    tunnel: [w508] -> w3
    tunnel: [w506] -> w2
    tunnel: [w505] -> w1
    tunnel: w7 -> [_]
    tunnel: w6 -> [_]
    tunnel: w5 -> [_]
    tunnel: w4 -> [_]
    tunnel: w3 -> [_]
    tunnel: w2 -> [_]
    tunnel: w1 -> [_]
    tunnel: [w518] -> _
    frame #0 {
      n170 = call <vilib>:"NI VeriStand - Close Workspace Manager Reference.vi"("WorkspaceManager"=w513) -> ("error out"=w512:errorcluster)  [unwired: 10 in]
      n171 = call <vilib>:"NI VeriStand - Close Engine State Change Notification.vi"("SystemStateRefs"=w514) -> ("error out"=w511:errorcluster)  [unwired: 10 in]
      n172 = Destroy User Event(user event=w516) -> (error out=w510:errorcluster)  [unwired: 1 in]
      n173 = Destroy User Event(user event=w517) -> (error out=w509:errorcluster)  [unwired: 1 in]
      n174 = Unregister For Events(event registration refnum=w515) -> (error out=w508:errorcluster)  [unwired: 1 in]
      n175 = call "STM Close Connection.vi"("connection info"=w507) -> ("error out"=w506:errorcluster)  [unwired: 10 in]
      n176 = Release Queue(queue=w504) -> (error out=w505:errorcluster)  [unwired: 2 in, 2 out]
    }
    frame #1 {
      n177 = invoke class="VI" method="FP.Close"() -> (error out=w518:errorcluster)  [unwired: 3 in, 2 out]
    }
  }
